vi "UICtrlsRefsAdd.vi"(8 "error in":errorcluster, 10 "UI Ctrl Refs":refnum<vi>[](array[refnum]), 11 "UI Ref cluster in":T1) -> (0 "error out":errorcluster, 3 "UI Ref cluster out":T1)   [LabVIEW 2025, in "UI_Library.lvlib" / "UI_Library.lvclass"]
doc: "Add new references to UI Cluster"
uses:
  UI_Library.lvclass
  Controls/UI_RefCluster.ctl
  <vilib>/Utility/Data Type/Type Definitions/Data Type.ctl
  <vilib>/Utility/Data Type/NI_Data Type.lvlib
  UI_Library.lvlib
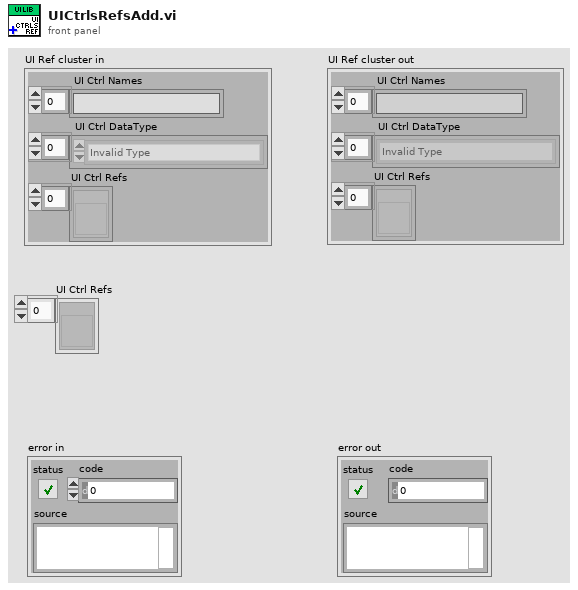
[diagram p1: front panel]
types:
  T1 = typedef "UI_Library.lvlib/UI_RefCluster.ctl" = cluster{"UI Ctrl Names":string[], "UI Ctrl DataType":T2[], "UI Ctrl Refs":refnum<vi>[]}
  T2 = typedef "NI_Data Type.lvlib/Data Type.ctl" = enum8{"Invalid Type", "Void", "I8", "I16", "I32", "I64", "U8", "U16", "U32", "U64", "Single Float", "Double Float", "Extended Float", "Single Complex", "Double Complex", "Extended Complex", "Enum U8", "Enum U16", "Enum U32", "Enum U64", "Single Float With Unit", "Double Float With Unit", "Extended Float With Unit", "Single Complex with Unit", "Double Complex with Unit", "Extended Complex with Unit", "Boolean", "String", "Path", "Picture", "Tag", "Array", "Cluster", "Variant", "LV Variant", "Waveform", "Timestamp", "Digital Waveform", "Digital Data", "ExpressData", "Refnum", "External Data", "VI", "Poly VI", "LabVIEW Class Instance", "Fixed Point", "Set Collection", "Map Collection"}
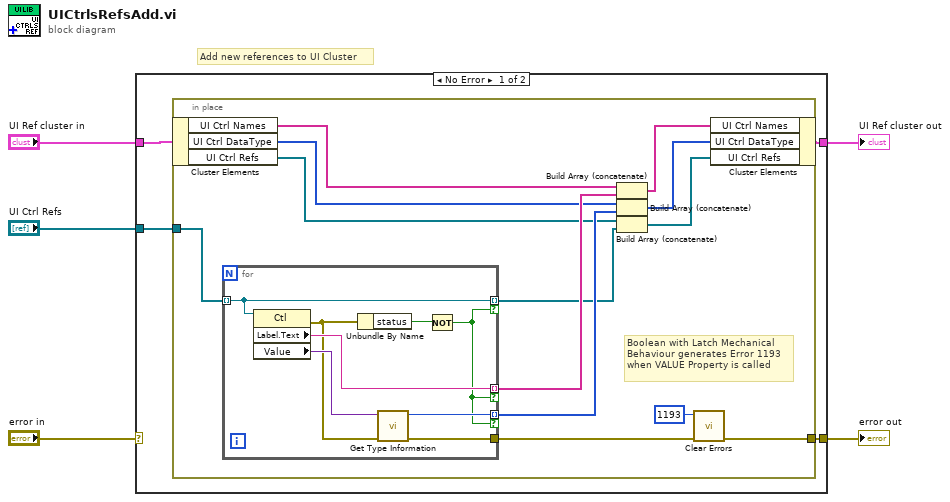
[diagram p0: block diagram]
diagram:
  # "Add new references to UI Cluster"
  n1 = case shown="No Error" "error in" {
    selector: "error in" -> [_ w32]
    tunnel: [w8 w32] -> w5
    tunnel: "UI Ref cluster in" -> [w7 w31]
    tunnel: [w6 w31] -> w3
    tunnel: "UI Ctrl Refs" -> [w9 _]
    frame No Error {
      n2 = in-place {
        in-place-border: w9 -> [w22]
        in-place-border: [w12] -> w8
        # "Boolean with Latch Mechanical\nBehaviour generates Error 1193 \nwhen VALUE Property is called"
        n3 = in-place-cluster #1(w7) -> ("UI Ctrl Names"=w18:string[], "UI Ctrl DataType"=w16:T2[], "UI Ctrl Refs"=w15:refnum<vi>[])
        n4 = for {
          tunnel: w22 -> [w26] mode=indexing
          tunnel: [w30] -> w21 mode=indexing if=w23
          tunnel: [w29] -> w20 mode=indexing if=w23
          tunnel: [w27] -> w19
          tunnel: [w26] -> w10 mode=indexing if=w23
          n5 = property class="Ctl"(reference=w26) -> (error out=w25:errorcluster, "Label.Text"=w30:string, "Value"=w28:variant)  [unwired: 1 in, 1 out]
          n6 = Unbundle By Name(w25) -> ("status"=w24:bool)
          n7 = call <vilib>:"Get Type Information.vi"("error in (no error)"=w25, "variant"=w28) -> ("error out"=w27:errorcluster, "type"=w29:T2)  [unwired: 5 in, 3 out]
          n8 = Not(x=w24) -> (.not. x?=w23:bool)
        }
        n9 = Build Array (concatenate)(w18, w21) -> (w17:string[])
        n10 = Build Array (concatenate)(w16, w20) -> (w14:T2[])
        n11 = Build Array (concatenate)(w15, w10) -> (w13:refnum<vi>[])
        n12 = call <vilib>:"Clear Errors.vi"("error in (no error)"=w19, "specific error code to clear (0: all)"=1193) -> ("error out"=w12:errorcluster)  [unwired: 4 in, 1 out]
        n13 = in-place-cluster #1("UI Ctrl Names"=w17, "UI Ctrl DataType"=w14, "UI Ctrl Refs"=w13) -> (w6:T1)
      }
    }
    frame Error {
    }
  }
  "error out" <- w5
  "UI Ref cluster out" <- w3
